vi "SVG2VSDX-command.vi"(8 "Error in":errorcluster caption="Error in (no error)", 10 "vsd路径":path, 11 "svg路径":path) -> (0 "Error out":errorcluster)   [LabVIEW 2018]
uses:
  Microsoft.Office.Interop.Visio
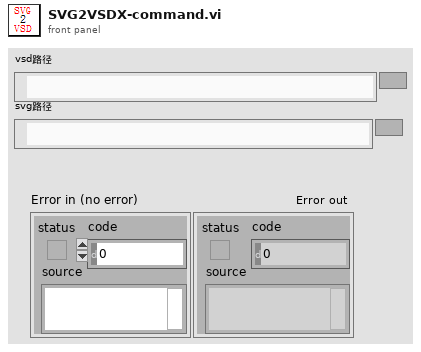
[diagram p1: front panel]
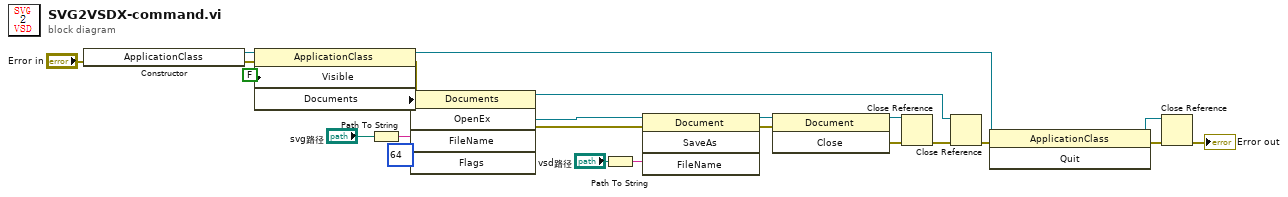
[diagram p0: block diagram]
diagram:
  n1 = constructor class="ApplicationClass"(error in="Error in") -> (reference out=w23:refnum<k24>, error out=w24:errorcluster)  [unwired: 2 in, 1 out]
  n2 = property on="属性节点" class="ApplicationClass"(reference=w23, error in=w24, "Visible"=FALSE) -> (reference out=w13:refnum<k24>, error out=w22:errorcluster, "Documents"=w12:refnum<k24>)
  n3 = Path To String(path="svg路径") -> (string=w18:string)
  n4 = invoke class="Documents" method="OpenEx"(reference=w12, error in=w22, "FileName"=w18, "Flags"=i16 64) -> (reference out=w21:refnum<k24>, error out=w20:errorcluster, "OpenEx"=w6:refnum<k24>)  [unwired: 1 in, 2 out]
  n5 = Path To String(path="vsd路径") -> (string=w15:string)
  n6 = invoke class="Document" method="SaveAs"(reference=w6, error in=w20, "FileName"=w15) -> (reference out=w19:refnum<k24>, error out=w8:errorcluster)  [unwired: 1 in, 2 out]
  n7 = invoke on="调用节点" class="Document" method="Close"(reference=w19, error in=w8) -> (reference out=w10:refnum<k24>, error out=w9:errorcluster)  [unwired: 1 in, 1 out]
  n8 = Close Reference(reference=w10, error in (no error)=w9) -> (error out=w5:errorcluster)
  n9 = Close Reference(reference=w21, error in (no error)=w5) -> (error out=w4:errorcluster)
  n10 = invoke on="调用节点" class="ApplicationClass" method="Quit"(reference=w13, error in=w4) -> (reference out=w7:refnum<k24>, error out=w3:errorcluster)  [unwired: 1 in, 1 out]
  n11 = Close Reference(reference=w7, error in (no error)=w3) -> (error out=→"Error out":errorcluster)
